vi "Model_Lifta.vi"() -> ()   [LabVIEW 2014]
panel:
  out "Grafik":dbl(graph)
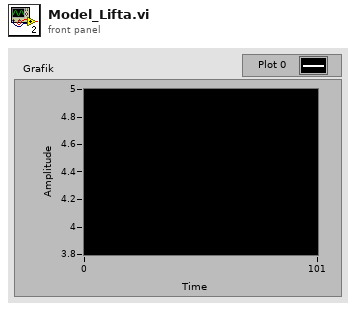
[diagram p1: front panel]
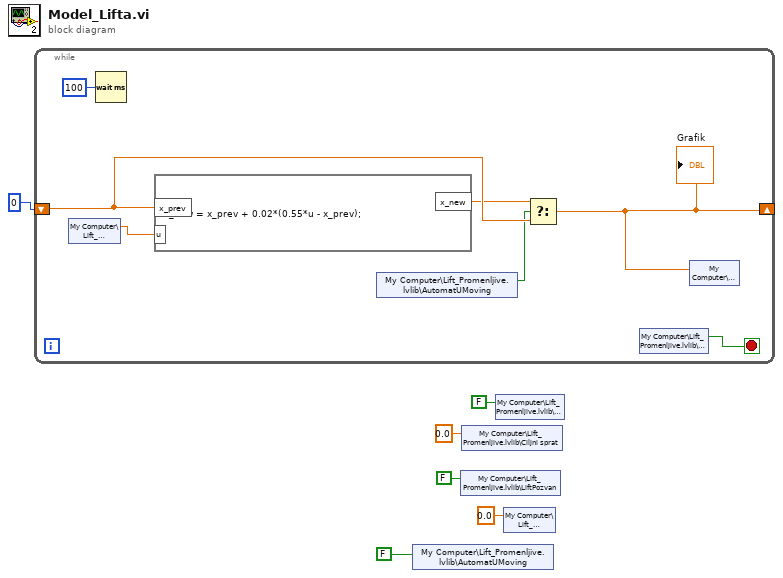
[diagram p0: block diagram]
diagram:
  n1 = while {
    shift-right: [w8] -> _
    shift-left: 0 -> [w12]
    stop <- w10 stop-if-true
    n2 = shared-variable "My Computer\\Lift_Promenljive.lvlib\\u"() -> (w7:dbl)  [unwired: 1 in, 1 out]
    n3 = Wait (ms)(milliseconds to wait=u32 100) -> ()  [unwired: 1 out]
    n4 = formula code="x_new = x_prev + 0.02*(0.55*u - x_prev);"("x_prev"=w12, "u"=w7) -> ("x_new"=w11:dbl)
    n5 = shared-variable "My Computer\\Lift_Promenljive.lvlib\\AutomatUMoving"() -> (w9:bool)  [unwired: 1 in, 1 out]
    n6 = Select(t=w11, s=w9, f=w12) -> (s? t:f=w8:dbl)
    "Grafik" <- w8
    n7 = shared-variable "My Computer\\Lift_Promenljive.lvlib\\Stop"() -> (w10:bool)  [unwired: 1 in, 1 out]
    n8 = shared-variable "My Computer\\Lift_Promenljive.lvlib\\x"(w8) -> ()  [unwired: 1 in, 1 out]
  }
  n9 = shared-variable "My Computer\\Lift_Promenljive.lvlib\\AutomatUMoving"(FALSE ("AutomatUMoving")) -> ()  [unwired: 1 in, 1 out]
  n10 = shared-variable "My Computer\\Lift_Promenljive.lvlib\\LiftPozvan"(FALSE ("LiftPozvan")) -> ()  [unwired: 1 in, 1 out]
  n11 = shared-variable "My Computer\\Lift_Promenljive.lvlib\\Ciljni sprat"(0.0 ("Ciljni sprat")) -> ()  [unwired: 1 in, 1 out]
  n12 = shared-variable "My Computer\\Lift_Promenljive.lvlib\\Stop"(FALSE ("Stop")) -> ()  [unwired: 1 in, 1 out]
  n13 = shared-variable "My Computer\\Lift_Promenljive.lvlib\\u"(0.0 ("u")) -> ()  [unwired: 1 in, 1 out]
